vi "sendStreamData.vi"(8 "error in (no error)":errorcluster, 10 "Stream data":string, 11 "SM1000-control in":T1) -> (0 "error out":errorcluster, 3 "SM1000-control out":T1)   [LabVIEW 2013, in "MaterialCharacterization.lvlib" / "MC-SM1000.lvclass"]
doc: "Send streaming data to an EC device session.\n\nMarking jobs are specified as sequences of data that represent instructions to the controller to set operational parameters, activate the laser steering galvos in both marking and non-marking modes, to interact with external devices, and to send event information back to a listening application. The job data is specified in an XML string, which is defined in the Streaming Job Data Definition section;\n\nJob execution by the controller starts as soon as the job data is received by the module and continues for as long as job data is available. Very large jobs can be partitioned into logical chunks, such as at marking object boundaries, and streamed out to the device as buffering on the host and target allow. Since the execution of the job and the process of streaming the data of the job are asynchronous and overlapped, it is possible to maintain continuous job execution with no pauses."
uses:
  MC-SM1000.lvclass
  Object-reference.ctl
  MC-SM1000.lvclass/MC-SM1000.ctl
  Custom-errors.ctl
  C:/Users/vangeste/Desktop/2015-06-02 - SLM - MAIF/HC-HardwareCharacterization/Sources/SM1000/LECSession.dll
  HC-HardwareCharacterization/Sources/SM1000/LECSession.dll
  DOTNET-error-int.vi
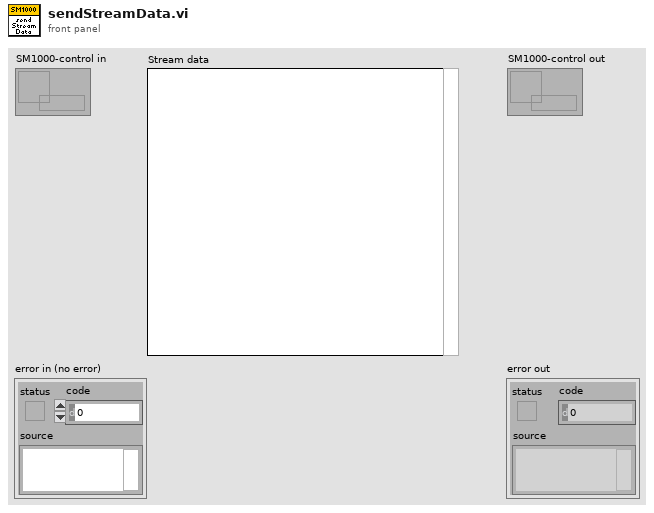
[diagram p1: front panel]
types:
  T1 = typedef "MaterialCharacterization.lvlib/MC-SM1000.lvclass/Object-reference.ctl" = refnum<data-value>
  T2 = typedef "MaterialCharacterization.lvlib/MC-SM1000.lvclass/Custom-errors.ctl" = enum16{"No error", "Not implemented", "Command not recognized", "Invalid input", "No connection", "Timeout", "Resource not loaded"}
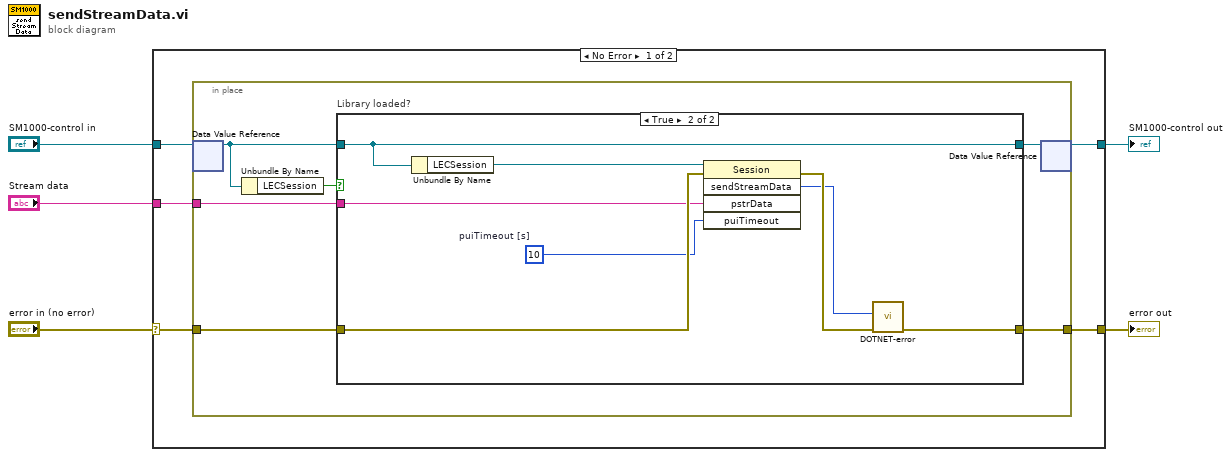
[diagram p0: block diagram]
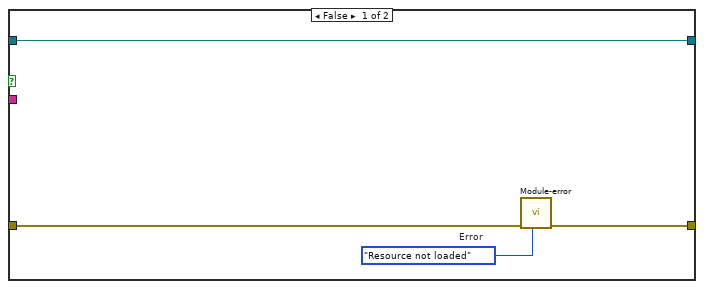
[diagram p2: hidden frame]
diagram:
  n1 = case shown="No Error" "error in (no error)" {
    selector: "error in (no error)" -> [w8 w30]
    tunnel: [w7 w30] -> w4
    tunnel: [w9 w29] -> w2
    tunnel: "SM1000-control in" -> [w10 w29]
    tunnel: "Stream data" -> [w6 _]
    frame No Error {
      n2 = in-place {
        in-place-border: w8 -> [w16]
        in-place-border: [w13] -> w7
        in-place-border: w6 -> [w11]
        n3 = in-place-dvr #1(w10) -> (w14:refnum<class "MC-SM1000.lvclass">)  [unwired: 1 out]
        n4 = Unbundle By Name(w14) -> ("LECSession"=w15:bool)
        n5 = case "Library loaded?" shown="True" w15 {
          tunnel: w16 -> [w20 w27]
          tunnel: w14 -> [w18 w26]
          tunnel: [w19 w23] -> w13
          tunnel: [w18 w26] -> w12
          tunnel: w11 -> [_ w25]
          frame False {
            w17 = Custom-errors."Resource not loaded"  # Error
            n6 = call "Module-error.vi"("Error"=w17, "error in (no error)"=w20) -> ("error out"=w19:errorcluster)  [unwired: 9 in]
          }
          frame True {
            w24 = u32 10  # puiTimeout [s]
            n7 = Unbundle By Name(w26) -> ("LECSession"=w28:refnum<k24>)
            n8 = invoke class="Session" method="sendStreamData"(reference=w28, error in=w27, "pstrData"=w25, "puiTimeout"=w24) -> (error out=w22:errorcluster, "sendStreamData"=w21:u32)  [unwired: 1 in, 3 out]
            n9 = call-poly "DOTNET-error.vi"("error in (no error)"=w22, "Retun code"=w21) -> ("error out"=w23:errorcluster)  [unwired: 9 in]
          }
        }
        n10 = in-place-dvr #1(w12) -> (w9:T1)  [unwired: 1 out]
      }
    }
    frame Error {
    }
  }
  "error out" <- w4
  "SM1000-control out" <- w2
